vi "SENS_SWE_SRCP_S.vi"(0 "VISA IN":refnum<visa-resource-name>, 1 "Source Power out Port1 or 2":i32, 5 "error in":errorcluster, 7 "Channel":i32) -> (14 "VISA Out":refnum<visa-resource-name>, 19 "error out":errorcluster)   [LabVIEW 2018, in "PNA-X.lvlib"]
doc: "SENSe<cnum>:SWEep:SRCPort <1 | 2> Superseded \nThis command is superseded. The Calc:Par:Def:Ext and Calc:Par:Mod:Ext can now optionally include the source \nport. \n(Read-Write) Sets the source port when making non S-parameter measurements. Has no effect on S-parameter \nmeasurements. \nParameters \n<cnum> Any existing channel number. If unspecified, value is set to 1 \n<1 | 2> 1 - Source power comes out Port 1 \n2 - Source power comes out Port 2 \nExamples SENS:SWE:SRCP 1 \nsense2:sweep:srcport 2 \nQuery Syntax SENSe<cnum>:SWEep:SRCPort? \n1818\n\nReturn Type Character \nDefault 1"
uses:
  PNA-X.lvlib
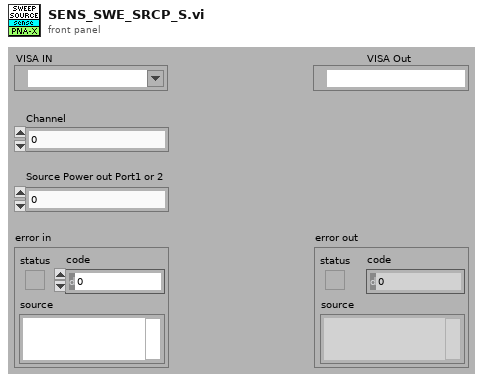
[diagram p1: front panel]
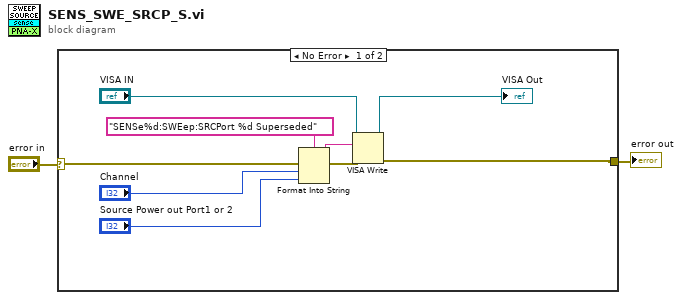
[diagram p0: block diagram]
diagram:
  n1 = case shown="No Error" "error in" {
    selector: "error in" -> [w11 w12]
    tunnel: [w6 w12] -> w1
    frame No Error {
      n2 = Format Into String(format string="SENSe%d:SWEep:SRCPort %d Superseded" ("Cmdline"), error in=w11, "Channel", "Source Power out Port1 or 2") -> (resulting string=w9:string, error out=w10:errorcluster)  [unwired: 1 in]
      n3 = VISA Write(VISA resource name="VISA IN", write buffer=w9, error in (no error)=w10) -> (VISA resource name out=→"VISA Out":refnum<visa-resource-name>, error out=w6:errorcluster)  [unwired: 1 out]
    }
    frame Error {
    }
  }
  "error out" <- w1
